vi "Graph_Builder.vi"(8 "Graph Data (array of clusters of XY Arrays)":cluster{"X2":dbl[], "Y2":dbl[]}[](array[cluster]), 9 "Index":i32, 10 "Y Point":dbl, 11 "X point":dbl) -> (0 "(XY Array) cluster out":cluster{"X2":dbl[], "Y2":dbl[]})   [LabVIEW 2019]
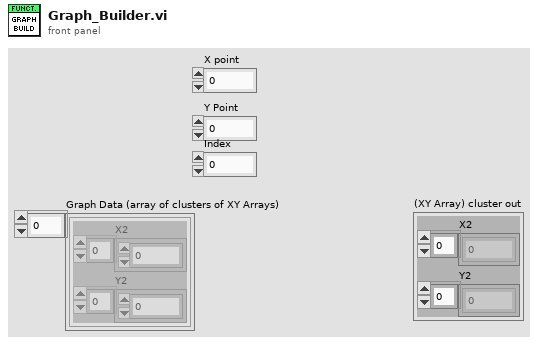
[diagram p1: front panel]
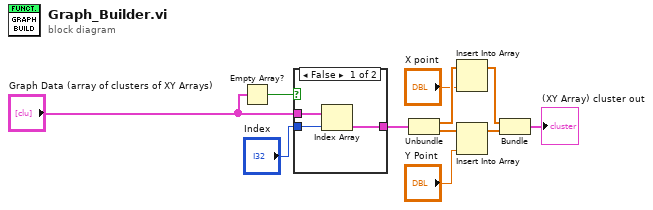
[diagram p0: block diagram]
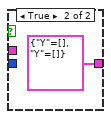
[diagram p2: hidden frame]
diagram:
  n1 = Empty Array?(array="Graph Data (array of clusters of XY Arrays)") -> (empty?=w2:bool)
  n2 = case shown="False" w2 {
    tunnel: "Graph Data (array of clusters of XY Arrays)" -> [w14 _]
    tunnel: "Index" -> [w13 _]
    tunnel: [w12 cluster{"Y":dbl[], "Y":dbl[]} {"Y"=[], "Y"=[]}] -> w4
    frame False {
      n3 = Index Array(array=w14, index=w13) -> (element=w12:cluster{"X2":dbl[], "Y2":dbl[]})
    }
    frame True {
    }
  }
  n4 = Unbundle(w4) -> ("Y"=w11:dbl[], "Y"=w10:dbl[])
  n5 = Insert Into Array(array=w11, new element="X point") -> (w9:dbl[])  [unwired: 1 in]
  n6 = Insert Into Array(array=w10, new element="Y Point") -> (w8:dbl[])  [unwired: 1 in]
  n7 = Bundle("Y"=w9, "Y"=w8) -> (→"(XY Array) cluster out":cluster{"Y":dbl[], "Y":dbl[]})  [unwired: 1 in]
